vi "Recipe.vi"() -> ()   [LabVIEW 2021]
panel:
  out "Recipe Complete":bool
  in  "Button 2":bool
  in  "Button":bool
  in  "Steps":string(tree)
  in  "Comment":string
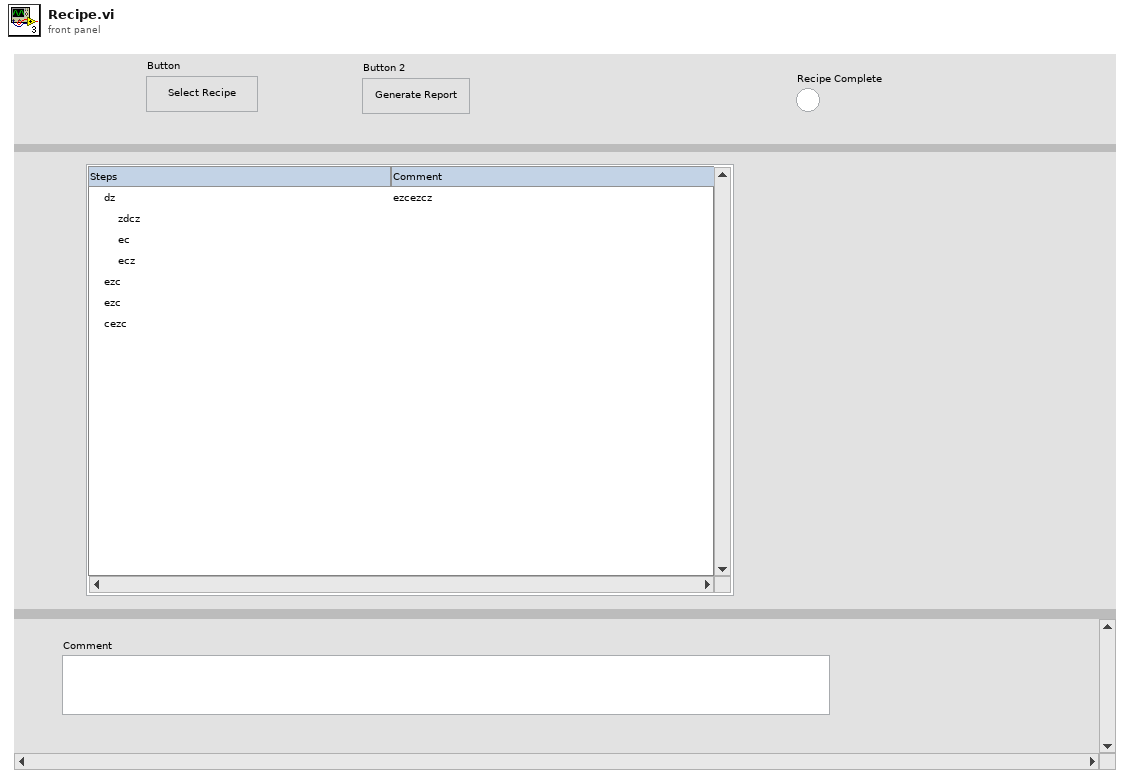
[diagram p1: front panel]
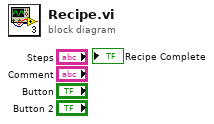
[diagram p0: block diagram]
diagram:
